vi "P-Thag.vi"(0 "Width":dbl, 3 "Length":dbl) -> (6 "Output":dbl)   [LabVIEW 2020]
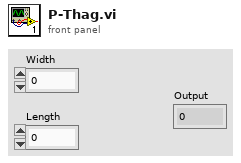
[diagram p1: front panel]
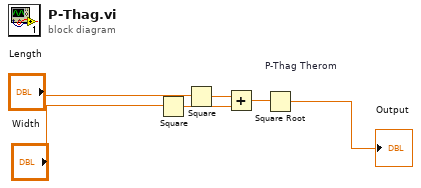
[diagram p0: block diagram]
diagram:
  n1 = Square(x="Width") -> (x^2=w4:dbl)
  n2 = Square(x="Length") -> (x^2=w3:dbl)
  n3 = Add(x=w3, y=w4) -> (x+y=w2:dbl)
  n4 = Square Root "P-Thag Therom"(x=w2) -> (sqrt(x)=→"Output":dbl)
